vi "Send InterDataCommunication_ZA.vi"(7 "Message Priority (Normal)":T2=enum."Normal", 8 "error in (no error)":errorcluster, 10 "InterDataCommunication_ZA":T1={"State Name"="Init", "Data"=variant}, 11 "Message Enqueuer":refnum<class "Message Enqueuer.lvclass">) -> (0 "error out":errorcluster, 3 "Message Enqueuer out":refnum<class "Message Enqueuer.lvclass">)   [LabVIEW 2019, in "Zen Analytics.lvlib" / "InterDataCommunication_ZA Msg.lvclass"]
doc: "This VI sends the message to an actor."
uses:
  InterDataCommunication_ZA Msg.lvclass
  <vilib>/ActorFramework/Message Enqueuer/Message Enqueuer.lvclass
  C:/Program Files/National Instruments/LabVIEW 2019/vi.lib/ActorFramework/Message/Message.lvclass
  <vilib>/ActorFramework/Message Enqueuer/Message Priority.ctl
  Zen Analytics/Dependency/InterDataCommunication.ctl
  Zen Analytics/Zen Analytics.lvclass
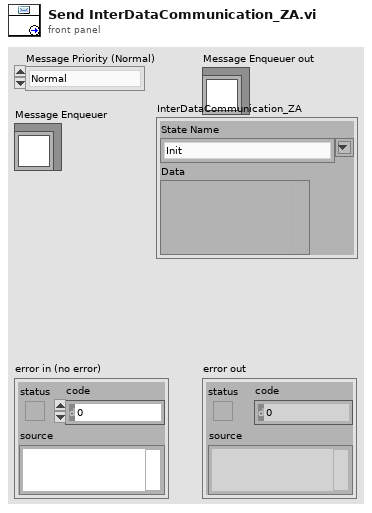
[diagram p1: front panel]
types:
  T1 = typedef "Zen Analytics.lvlib/Zen Analytics.lvclass/InterDataCommunication.ctl" = cluster{"State Name":string, "Data":variant}
  T2 = typedef "Actor Framework.lvlib/Message Enqueuer.lvclass/Message Priority.ctl" = enum16{"Low", "Normal", "High"}
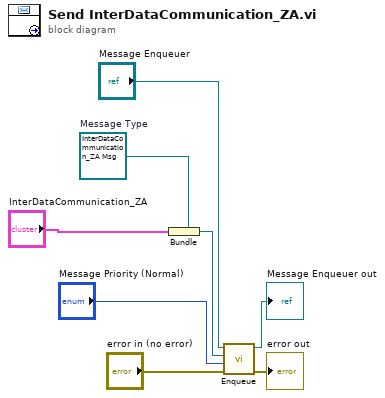
[diagram p0: block diagram]
diagram:
  w5 = refnum<class "InterDataCommunication_ZA Msg.lvclass"> refnum  # Message Type
  n1 = Bundle(cluster=w5, "InterDataCommunication_ZA") -> (w4:refnum<class "InterDataCommunication_ZA Msg.lvclass">)
  n2 = call <vilib>:"Enqueue.vi"("error in (no error)"="error in (no error)", "Message Priority (Normal)"="Message Priority (Normal)", "Message"=w4, "Message Enqueuer in"="Message Enqueuer") -> ("error out"=→"error out":errorcluster, "Message Enqueuer out"=→"Message Enqueuer out":refnum<class "Message Enqueuer.lvclass">)  [unwired: 6 in]
